vi "Transmit Datagram.vi"(5 "transfer id":i32, 7 "transfer group id":i32, 8 "error in (no error)":errorcluster, 9 "transfer data":string, 11 "UDP Transceiver in":refnum<class "UDP Transceiver.lvclass">) -> (0 "error out":errorcluster, 3 "UDP Transceiver out":refnum<class "UDP Transceiver.lvclass">)   [LabVIEW 2017, in "UDP.lvlib" / "UDP Transceiver.lvclass"]
uses:
  UDP Transceiver.lvclass
  UDP Transceiver.lvclass/UDP Transceiver.ctl
  <vilib>/Utility/error.llb/Clear Errors.vi
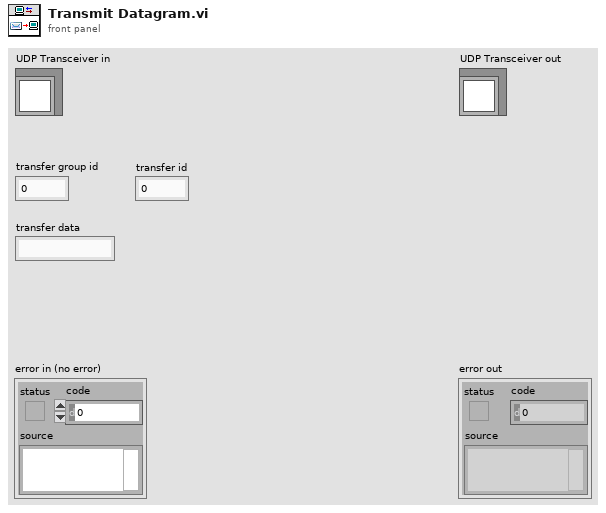
[diagram p1: front panel]
types:
  T1 = typedef "UDP.lvlib/UDP Transceiver.lvclass/Transfer Group Parameters.ctl" = cluster{"transfers":T2[], "max size":i32, "timeout":i32}
  T2 = typedef "UDP.lvlib/UDP Transceiver.lvclass/Transfer Parameters.ctl" = cluster{"group offset":u64, "size":u64, "address":u32, "port":u16}
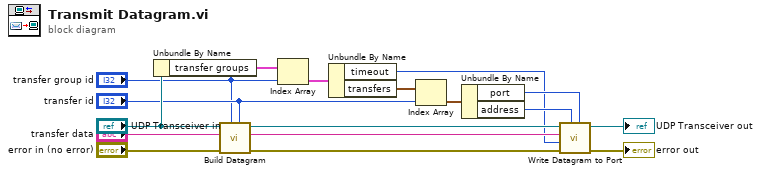
[diagram p0: block diagram]
diagram:
  n1 = Unbundle By Name("UDP Transceiver in") -> ("transfer groups"=w9:T1[])
  n2 = call-dynamic "Build Datagram.vi"("transfer id"="transfer id", "transfer group id"="transfer group id", "error in (no error)"="error in (no error)", "transfer data"="transfer data", "UDP Transceiver in"="UDP Transceiver in") -> ("error out"=w13:errorcluster, "datagram"=w14:string, "UDP Transceiver out"=w10:refnum<class "UDP Transceiver.lvclass">)  [unwired: 4 in]
  n3 = Index Array(array=w9, index="transfer group id") -> (element=w8:T1)
  n4 = Unbundle By Name(w8) -> ("timeout"=w1:i32, "transfers"=w6:T2[])
  n5 = Index Array(array=w6, index="transfer id") -> (element=w7:T2)
  n6 = Unbundle By Name(w7) -> ("port"=w2:u16, "address"=w3:u32)
  n7 = call "Write Datagram to Port.vi"("destination port"=w2, "destination address"=w3, "error in (no error)"=w13, "timeout ms (25000)"=w1, "data"=w14, "UDP Transceiver in"=w10) -> ("error out"=→"error out":errorcluster, "UDP Transceiver out"=→"UDP Transceiver out":refnum<class "UDP Transceiver.lvclass">)  [unwired: 3 in, 1 out]
